vi "DBC_Create_Signal_Entry.vi"(5 "Name Cluster":cluster{"Name":T1, "Comment":T1}, 6 "Config":T2={"Index"=0, "Start Bit"=0, "Data Type"=0, "Number of Bits"=32} {"Data Type" items=["Signed", "Unsigned", "IEEE Float", "Byte Array"]}, 7 "Status Scale":sgl[](array[numeric]), 8 "Fehler (Eingang, kein Fehler)":errorcluster, 9 "Optionsfelder Status":T3(ring), 10 "Scale overall":sgl, 11 "Frame (Eingang)":refnum<k21>) -> (0 "Fehler (Ausgang)":errorcluster, 2 "Scale overall out":sgl, 3 "Referenz (Ausgang)":refnum<k21>)   [LabVIEW 2020, in "CAN Konfig.lvlib"]
uses:
  SAE J-1939 SignalConfig.ctl
  Visualisierungs Elemente/String - Ausgabefeld.ctl
  <vilib>/xnet/xnet.llb/XNET Database Create (Signal).vi
  CAN Konfig.lvlib
  <resource>/objmgr/xnet.rc
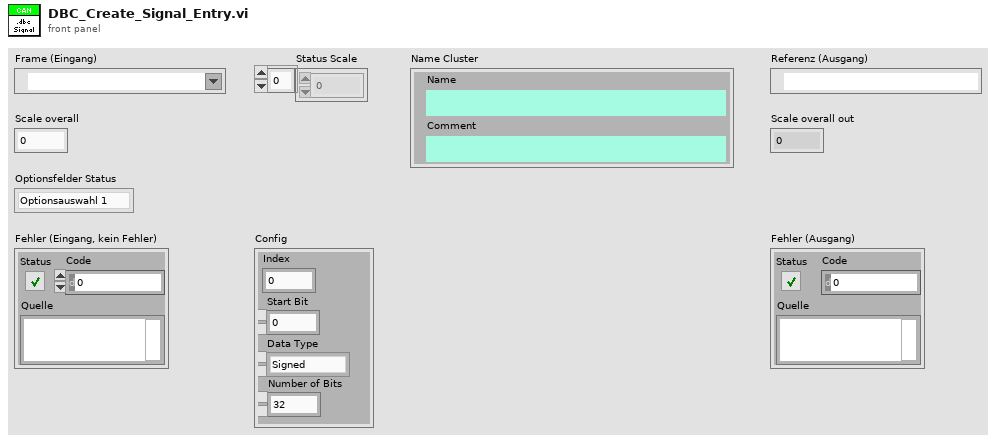
[diagram p1: front panel]
types:
  T1 = typedef "String - Ausgabefeld.ctl" = string
  T2 = typedef "CAN Konfig.lvlib/SAE J-1939 SignalConfig.ctl" = cluster{"Index":i32, "Start Bit":u32, "Data Type":u32, "Number of Bits":u32}
  T3 = enum32{"Optionsauswahl 1", "Optionsauswahl 2", "Optionsauswahl 3"}
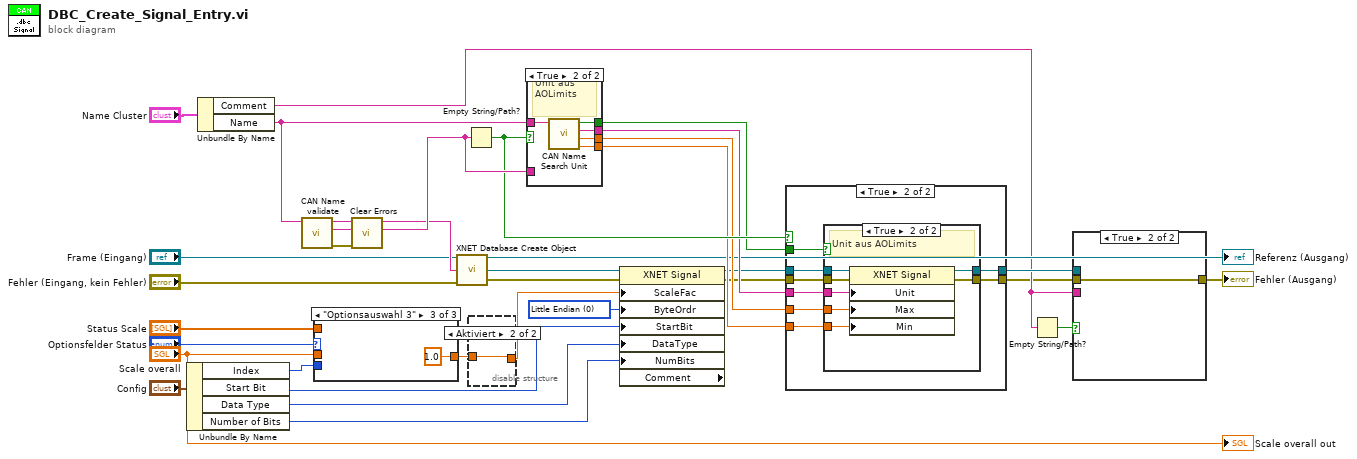
[diagram p0: block diagram]
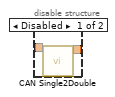
[diagram p2: hidden frame]
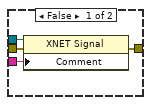
[diagram p3: hidden frame]
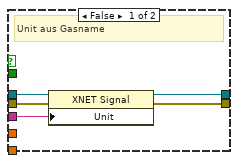
[diagram p5: hidden frame]
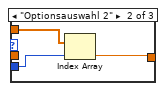
[diagram p8: hidden frame]
diagram:
  w11 = u32 0 items=["Little Endian", "Big Endian"] ("Byte Order")
  n1 = Unbundle By Name("Config") -> ("Index"=w15:i32, "Start Bit"=w14:u32, "Data Type"=w13:u32, "Number of Bits"=w10:u32)
  n2 = Unbundle By Name("Name Cluster") -> ("Comment"=w5:T1, "Name"=w8:T1)
  n3 = call "CAN Name validate.vi"("Gas Name in"=w8) -> ("error out"=w12:errorcluster, "found Unit out"=w33:T1, "valid Name out"=w32:T1)  [unwired: 8 in]
  n4 = case shown="\"Optionsauswahl 3\"" "Optionsfelder Status" {
    tunnel: "Scale overall" -> [w34 _ _]
    tunnel: [w34 w35 sgl 1.0] -> w22
    tunnel: "Status Scale" -> [_ w37 _]
    tunnel: w15 -> [_ w36 _]
    frame "Optionsauswahl 1", Default {
    }
    frame "Optionsauswahl 2" {
      n5 = Index Array(array=w37, index=w36) -> (element=w35:sgl)
    }
    frame "Optionsauswahl 3" {
    }
  }
  n6 = call <vilib>:"Clear Errors.vi"("error in (no error)"=w12) -> ()  [unwired: 5 in, 2 out]
  n7 = call-poly <vilib>:"XNET Database Create Object.vi"("frame in"="Frame (Eingang)", "signal name"=w32, "error in (no error)"="Fehler (Eingang, kein Fehler)") -> ("frame out"=→"Referenz (Ausgang)":refnum<k21>, "signal out"=w17:refnum<k21>, "error out"=w18:errorcluster)  [unwired: 10 in]
  n8 = Empty String/Path?(string/path=w33) -> (empty?=w31:bool)
  n9 = disable-structure shown="Aktiviert" {
    disable-tunnel: w22 -> [w40 w41]
    disable-tunnel: [w39 w41] -> w1
    frame Disabled {
      n10 = call "CAN Single2Double.vi"("Scale overall"=w40) -> ("Numerisch"=w39:dbl)  [unwired: 9 in, 1 out]
    }
    frame Enabled {
    }
  }
  n11 = case shown="True" w31 {
    tunnel: w33 -> [w42 _]
    tunnel: w8 -> [_ w47]
    tunnel: [_ w46] -> w27
    tunnel: [w42 w45] -> w28
    tunnel: [_ w44] -> w30
    tunnel: [_ w43] -> w29
    frame False {
    }
    frame True {
      # "Unit aus AOLimits"
      n12 = call "CAN Name Search Unit.vi"("Gas Name"=w47) -> ("Min"=w43:dbl, "Max"=w46:dbl, "Unit"=w45:string, "Gefunden?"=w44:bool)  [unwired: 7 in]
    }
  }
  n13 = property class="XNET Signal" props=["ScaleFac", "ByteOrdr", "StartBit", "DataType", "NumBits", "Comment"](reference=w17, error in=w18, "ScaleFac"=w1, "ByteOrdr"=w11, "StartBit"=w14, "DataType"=w13, "NumBits"=w10) -> (reference out=w26:refnum<k21>, error out=w25:errorcluster)  [unwired: 1 out]
  n14 = case shown="True" w31 {
    tunnel: [w52 w60] -> w4
    tunnel: w25 -> [w51 w59]
    tunnel: w26 -> [w50 w58]
    tunnel: w29 -> [_ w57]
    tunnel: w27 -> [_ w56]
    tunnel: w28 -> [w49 w55]
    tunnel: w30 -> [_ w54]
    tunnel: [w48 w53] -> w6
    frame False {
      # "Unit aus Gasname"
      n15 = property class="XNET Signal"(reference=w50, error in=w51, "Unit"=w49) -> (reference out=w48:refnum<k21>, error out=w52:errorcluster)
    }
    frame True {
      n16 = case shown="True" w54 {
        tunnel: [w62 w69] -> w60
        tunnel: w59 -> [w62 w68]
        tunnel: w58 -> [w61 w67]
        tunnel: w57 -> [_ w66]
        tunnel: w56 -> [_ w65]
        tunnel: w55 -> [_ w64]
        tunnel: [w61 w63] -> w53
        frame False {
        }
        frame True {
          # "Unit aus AOLimits"
          n17 = property class="XNET Signal"(reference=w67, error in=w68, "Unit"=w64, "Max"=w65, "Min"=w66) -> (reference out=w63:refnum<k21>, error out=w69:errorcluster)
        }
      }
    }
  }
  n18 = Empty String/Path?(string/path=w5) -> (empty?=w7:bool)
  n19 = case shown="True" w7 {
    tunnel: w6 -> [w73 _]
    tunnel: w5 -> [w72 _]
    tunnel: w4 -> [w71 w74]
    tunnel: [w70 w74] -> w3
    frame False {
      n20 = property class="XNET Signal"(reference=w73, error in=w71, "Comment"=w72) -> (error out=w70:errorcluster)  [unwired: 1 out]
    }
    frame True {
    }
  }
  "Fehler (Ausgang)" <- w3
  "Scale overall out" <- "Scale overall"
